vi "Trigger.vi"(8 "error in (no error)":errorcluster, 11 "Micron sm Digitizer in":refnum<class "Micron sm Digitizer.lvclass">) -> (0 "error out":errorcluster, 3 "Micron sm Digitizer out":refnum<class "Micron sm Digitizer.lvclass">)   [LabVIEW 2024, in "Micron sm Digitizer.lvclass"]
uses:
  Micron sm Digitizer.lvclass
  Micron sm Digitizer.lvclass/Micron sm Digitizer.ctl
  Micron Optics sm130/Micron Optics sm130.lvlib
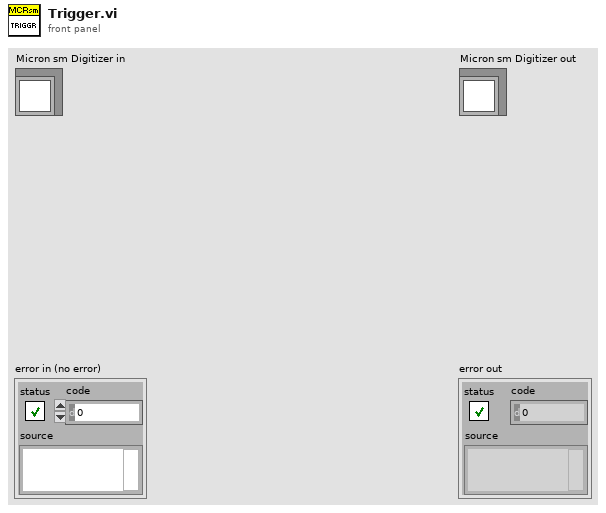
[diagram p1: front panel]
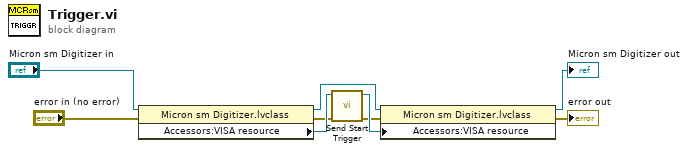
[diagram p0: block diagram]
diagram:
  n1 = property class="Micron sm Digitizer.lvclass"(reference="Micron sm Digitizer in", error in="error in (no error)") -> (reference out=w5:refnum<class "Micron sm Digitizer.lvclass">, error out=w2:errorcluster, "Accessors:VISA resource"=w3:refnum<visa-resource-name>)
  n2 = call "Send Start Trigger.vi"("error in (no error)"=w2, "VISA resource name"=w3) -> ("error out"=w1:errorcluster, "VISA resource name out"=w4:refnum<visa-resource-name>)  [unwired: 8 in]
  n3 = property class="Micron sm Digitizer.lvclass"(reference=w5, error in=w1, "Accessors:VISA resource"=w4) -> (reference out=→"Micron sm Digitizer out":refnum<class "Micron sm Digitizer.lvclass">, error out=→"error out":errorcluster)
